vi "PID Ziegler-Nichols Table.vi"(6 "Ziegler-Nichlos Speed":u16(ring) items=["Fast", "Normal", "Slow"], 7 "Type of Controller":u16(ring) items=["P", "PI", "PID"], 9 "Dead Time (L)":dbl, 10 "Time Constant (T)":dbl, 11 "Plant Gain (K)":dbl) -> (1 "Derivative Time (Td)":dbl, 2 "Integral Time (Ti)":dbl, 3 "Proportional Gain (Kp)":dbl)   [LabVIEW 2020, in "NI_PID_autopid.lvlib"]
uses:
  <vilib>/addons/control/pid/NI_PID_autopid.lvlib
panel:
  out "Kp 6":dbl
  out "Kp 5":dbl
  out "Kp 4":dbl
  out "Kp 3":dbl
  out "Kp 2":dbl
  out "Kp":dbl
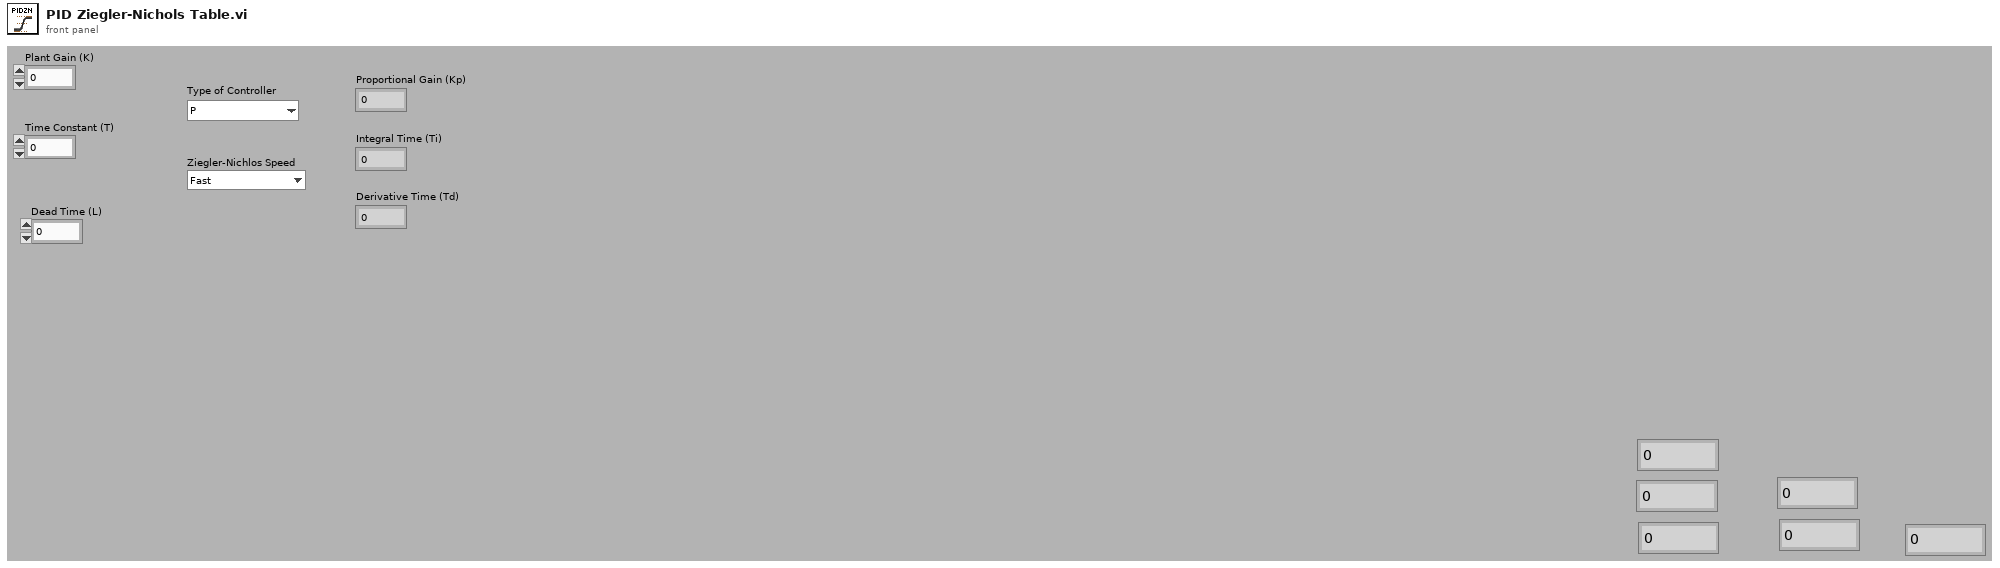
[diagram p1: front panel]
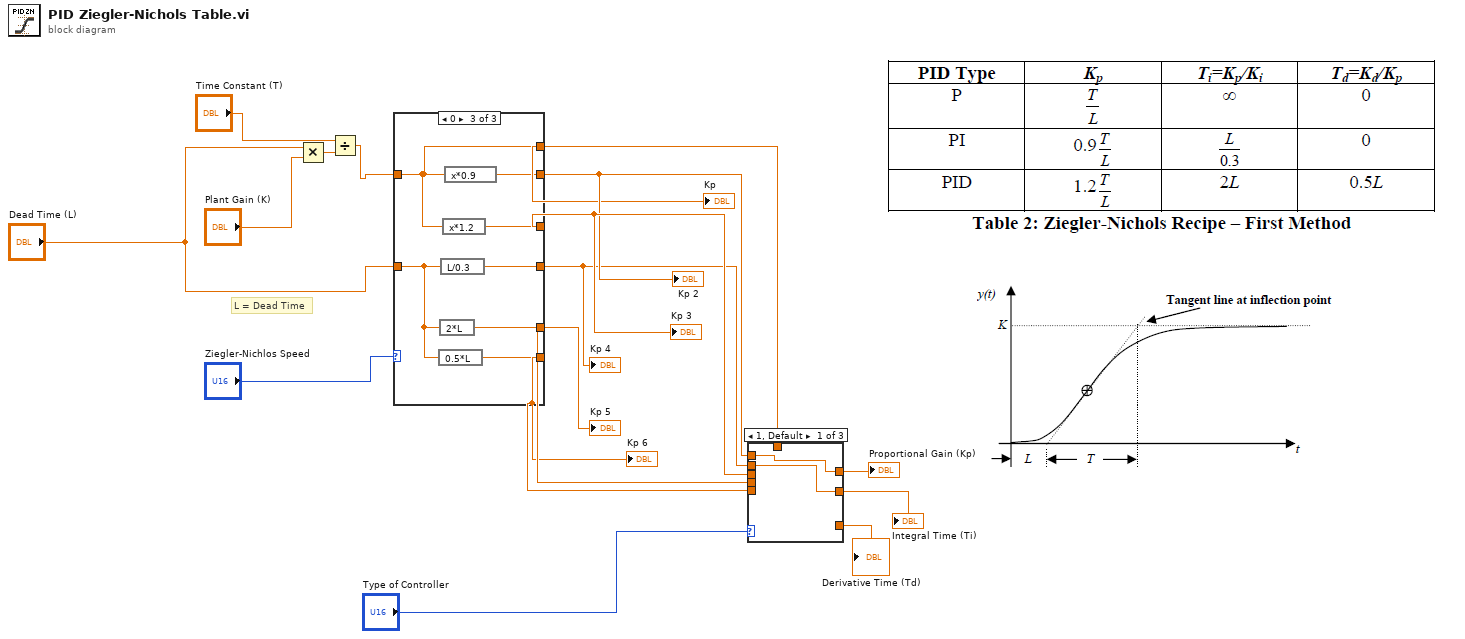
[diagram p0: block diagram]
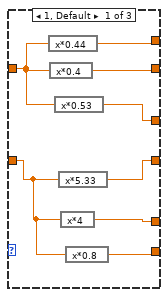
[diagram p2: hidden frame]
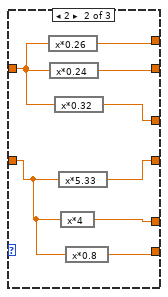
[diagram p3: hidden frame]
diagram:
  # "L = Dead Time"
  n1 = Multiply(x="Dead Time (L)", y="Plant Gain (K)") -> (x*y=w15:dbl)
  n2 = Divide(x="Time Constant (T)", y=w15) -> (x/y=w7:dbl)
  n3 = case shown="0" "Ziegler-Nichlos Speed" {
    tunnel: "Dead Time (L)" -> [w18 w26 w39]
    tunnel: [w21 w29 w38] -> w13
    tunnel: [w19 w27 w37] -> w12
    tunnel: [w17 w25 w36] -> w11
    tunnel: w7 -> [w22 w30 w33]
    tunnel: [w23 w31 w35] -> w10
    tunnel: [w20 w28 w34] -> w9
    tunnel: [w24 w32 w33] -> w8
    frame 1, Default {
      n4 = expression code="x*0.44"(w22) -> (w24:dbl)
      n5 = expression code="x*0.4"(w22) -> (w23:dbl)
      n6 = expression code="x*0.53"(w22) -> (w21:dbl)
      n7 = expression code="x*5.33"(w18) -> (w20:dbl)
      n8 = expression code="x*4"(w18) -> (w19:dbl)
      n9 = expression code="x*0.8"(w18) -> (w17:dbl)
    }
    frame 2 {
      n10 = expression code="x*0.26"(w30) -> (w32:dbl)
      n11 = expression code="x*0.24"(w30) -> (w31:dbl)
      n12 = expression code="x*0.32"(w30) -> (w29:dbl)
      n13 = expression code="x*5.33"(w26) -> (w28:dbl)
      n14 = expression code="x*4"(w26) -> (w27:dbl)
      n15 = expression code="x*0.8"(w26) -> (w25:dbl)
    }
    frame 0 {
      n16 = expression code="0.5*L"(w39) -> (w36:dbl)
      n17 = expression code="2*L"(w39) -> (w37:dbl)
      n18 = expression code="L/0.3"(w39) -> (w34:dbl)
      n19 = expression code="x*1.2"(w33) -> (w38:dbl)
      n20 = expression code="x*0.9"(w33) -> (w35:dbl)
    }
  }
  "Kp" <- w8
  "Kp 2" <- w10
  "Kp 3" <- w13
  "Kp 4" <- w9
  "Kp 5" <- w12
  "Kp 6" <- w11
  n21 = case shown="1, Default" "Type of Controller" {
    tunnel: w13 -> [_ _ w45]
    tunnel: w12 -> [_ _ w44]
    tunnel: w11 -> [_ _ w43]
    tunnel: w8 -> [_ w42 _]
    tunnel: w10 -> [w40 _ _]
    tunnel: w9 -> [w41 _ _]
    tunnel: [w40 w42 w45] -> w4
    tunnel: [w41 _ w44] -> w3
    tunnel: [_ _ w43] -> w2
    frame 1, Default {
    }
    frame 0 {
    }
    frame 2 {
    }
  }
  "Proportional Gain (Kp)" <- w4
  "Integral Time (Ti)" <- w3
  "Derivative Time (Td)" <- w2
